vi "close.vi"(8 "error in":errorcluster, 11 "Profibus Module runtime in":refnum<class "Profibus Module runtime.lvclass">) -> (0 "error out":errorcluster)   [LabVIEW 2013, in "Profibus Module runtime.lvclass"]
doc: "Provides an interface for terminating a module instance. While this interface performs no operations, a child should close and deallocate any open references or memory."
uses:
  Profibus Module runtime.lvclass
  Profibus Module runtime.lvclass/Profibus Module runtime.ctl
  dynamic profibus/dynamic profibus.lvlib
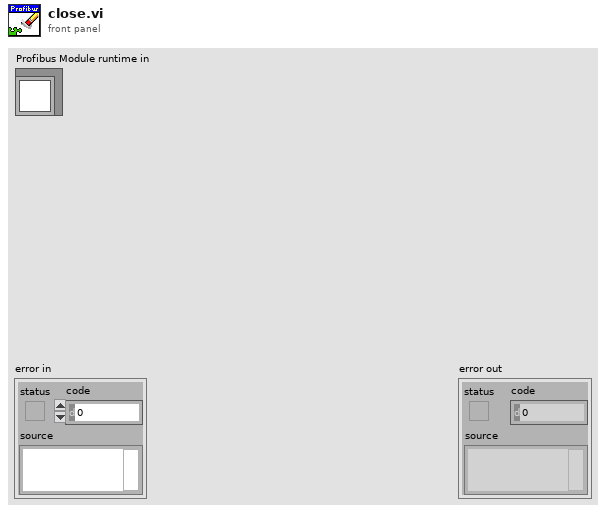
[diagram p1: front panel]
types:
  T1 = typedef "dynamic profibus.lvlib/fpga reference.ctl" = refnum<k20>
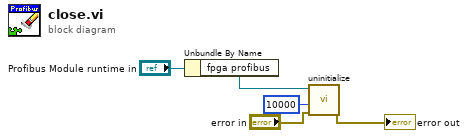
[diagram p0: block diagram]
diagram:
  n1 = Unbundle By Name("Profibus Module runtime in") -> ("fpga profibus"=w2:T1)
  n2 = call "uninitialize.vi"("error in"="error in", "Timeout (ms)"=10000, "profibus reference"=w2) -> ("error out"=→"error out":errorcluster)  [unwired: 7 in, 1 out]
